vi "V1.0.vi"() -> ()   [LabVIEW 2019]
uses:
  subVI/move/position cluster.ctl
panel:
  out "error out":errorcluster
  in  "Position in":T1
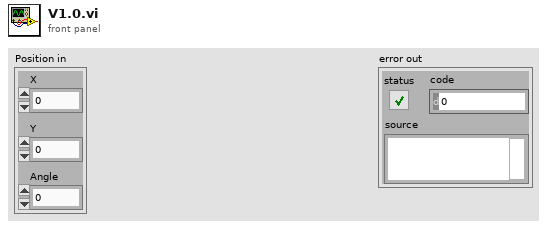
[diagram p1: front panel]
types:
  T1 = typedef "position cluster.ctl" = cluster{"X":dbl, "Y":dbl, "Angle":dbl}
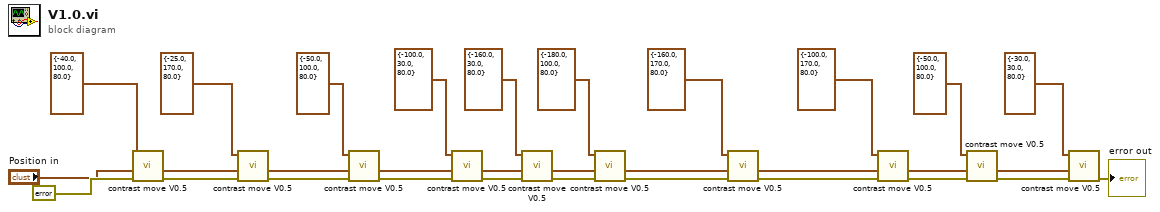
[diagram p0: block diagram]
diagram:
  n1 = call "contrast move V0.5.vi"("error in (no error)"=errorcluster {"status"=FALSE, "code"=0, "source"=""}, "Position in"="Position in", "Target position"=cluster{"X":dbl, "Y":dbl, "speed":dbl} {"X"=-40.0, "Y"=100.0, "speed"=80.0}) -> ("error out"=w28:errorcluster, "Position out"=w27:T1)  [unwired: 7 in]
  n2 = call "contrast move V0.5.vi"("error in (no error)"=w28, "Position in"=w27, "Target position"=cluster{"X":dbl, "Y":dbl, "speed":dbl} {"X"=-25.0, "Y"=170.0, "speed"=80.0}) -> ("error out"=w25:errorcluster, "Position out"=w24:T1)  [unwired: 7 in]
  n3 = call "contrast move V0.5.vi"("error in (no error)"=w25, "Position in"=w24, "Target position"=cluster{"X":dbl, "Y":dbl, "speed":dbl} {"X"=-50.0, "Y"=100.0, "speed"=80.0}) -> ("error out"=w22:errorcluster, "Position out"=w21:T1)  [unwired: 7 in]
  n4 = call "contrast move V0.5.vi"("error in (no error)"=w22, "Position in"=w21, "Target position"=cluster{"X":dbl, "Y":dbl, "speed":dbl} {"X"=-100.0, "Y"=30.0, "speed"=80.0}) -> ("error out"=w18:errorcluster, "Position out"=w17:T1)  [unwired: 7 in]
  n5 = call "contrast move V0.5.vi"("error in (no error)"=w18, "Position in"=w17, "Target position"=cluster{"X":dbl, "Y":dbl, "speed":dbl} {"X"=-160.0, "Y"=30.0, "speed"=80.0}) -> ("error out"=w15:errorcluster, "Position out"=w14:T1)  [unwired: 7 in]
  n6 = call "contrast move V0.5.vi"("error in (no error)"=w15, "Position in"=w14, "Target position"=cluster{"X":dbl, "Y":dbl, "speed":dbl} {"X"=-180.0, "Y"=100.0, "speed"=80.0}) -> ("error out"=w12:errorcluster, "Position out"=w11:T1)  [unwired: 7 in]
  n7 = call "contrast move V0.5.vi"("error in (no error)"=w12, "Position in"=w11, "Target position"=cluster{"X":dbl, "Y":dbl, "speed":dbl} {"X"=-160.0, "Y"=170.0, "speed"=80.0}) -> ("error out"=w8:errorcluster, "Position out"=w9:T1)  [unwired: 7 in]
  n8 = call "contrast move V0.5.vi"("error in (no error)"=w8, "Position in"=w9, "Target position"=cluster{"X":dbl, "Y":dbl, "speed":dbl} {"X"=-100.0, "Y"=170.0, "speed"=80.0}) -> ("error out"=w5:errorcluster, "Position out"=w6:T1)  [unwired: 7 in]
  n9 = call "contrast move V0.5.vi"("error in (no error)"=w5, "Position in"=w6, "Target position"=cluster{"X":dbl, "Y":dbl, "speed":dbl} {"X"=-50.0, "Y"=100.0, "speed"=80.0}) -> ("error out"=w4:errorcluster, "Position out"=w3:T1)  [unwired: 7 in]
  n10 = call "contrast move V0.5.vi"("error in (no error)"=w4, "Position in"=w3, "Target position"=cluster{"X":dbl, "Y":dbl, "speed":dbl} {"X"=-30.0, "Y"=30.0, "speed"=80.0}) -> ("error out"=→"error out":errorcluster)  [unwired: 7 in, 1 out]
